vi "复件 终止项.vi"(1 "结果":i32[][](array[numeric]), 2 "检索":i32[][](array[numeric])) -> (0 "结果 2":i32[][](array[numeric]))   [LabVIEW 2014]
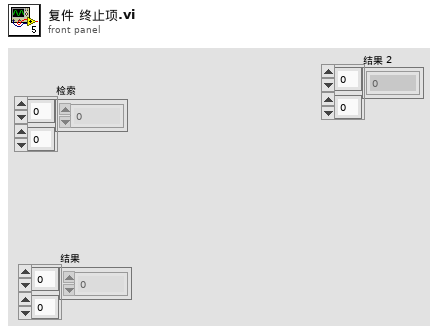
[diagram p1: front panel]
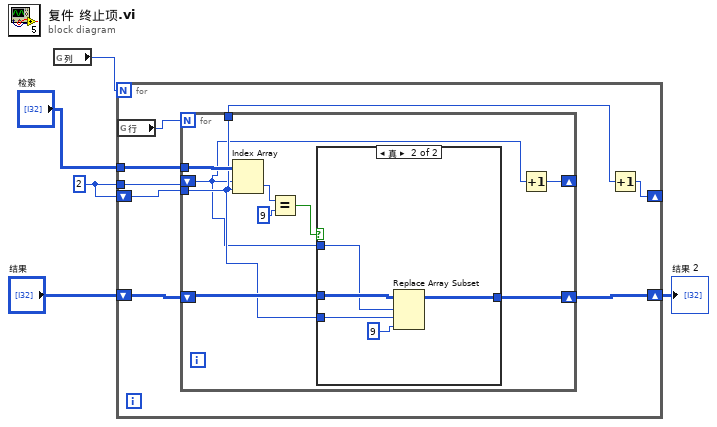
[diagram p0: block diagram]
diagram:
  w4 = 2
  n1 = global read "全局 1.vi" "列"() -> (w3:i32)
  n2 = for {
    N: w3 -> [_]
    tunnel: "检索" -> [w13]
    tunnel: w4 -> [w11]
    shift-right: [w10] -> _
    shift-left: w4 -> [w9]
    shift-right: [w7] -> w1
    shift-left: "结果" -> [w6]
    n3 = global read "全局 1.vi" "行"() -> (w8:i32)
    n4 = for {
      N: w8 -> [_]
      tunnel: w13 -> [w22]
      tunnel: w9 -> [w15]
      shift-right: [w18] -> _
      shift-left: w11 -> [w14]
      tunnel: [w15] -> w12
      shift-right: [w17] -> w7
      shift-left: w6 -> [w16]
      n5 = Index Array(array=w22, index (row)=w14, index (col)=w15) -> (element=w21:i32)
      n6 = Equal?(x=w21, y=9) -> (x = y?=w19:bool)
      n7 = case shown="真" w19 {
        tunnel: w16 -> [w23 w28]
        tunnel: [w23 w27] -> w17
        tunnel: w15 -> [_ w26]
        tunnel: w14 -> [_ w25]
        frame False {
        }
        frame True {
          n8 = Replace Array Subset(array=w28, new element=9, index (row)=w25, index (col)=w26) -> (w27:i32[][])
        }
      }
      n9 = Increment(x=w14) -> (x+1=w18:i32)
    }
    n10 = Increment(x=w12) -> (x+1=w10:i32)
  }
  "结果 2" <- w1
